vi "Menu Refs.vi"(8 "error in":errorcluster, 10 "Disabled 2":T1(ring), 11 "ATM Data":T2={"UI Refs"={"Right Buttons"=refnum, "Left Buttons"=refnum, "User Input"=refnum, "ATM Messages"=refnum, "Left Menu"=refnum, "Right Menu"=refnum, "Enter"=refnum}, "Map"={}, "Login Valid?"=FALSE, "Queue Message"=refnum, "State"=enum."None", "User"={"Pin"="", "First Name"="", "Last Name"="", "Balance"=0.0, "Login Valid?"=FALSE}, "Main States"={"Message"="Initialize", "Data"=variant}}) -> (0 "error out":errorcluster, 3 "ATM Data Out":T2={"UI Refs"={"Right Buttons"=refnum, "Left Buttons"=refnum, "User Input"=refnum, "ATM Messages"=refnum, "Left Menu"=refnum, "Right Menu"=refnum, "Enter"=refnum}, "Map"={}, "Login Valid?"=FALSE, "Queue Message"=refnum, "State"=enum."None", "User"={"Pin"="", "First Name"="", "Last Name"="", "Balance"=0.0, "Login Valid?"=FALSE}, "Main States"={"Message"="Initialize", "Data"=variant}})   [LabVIEW 2020, in "ATM Machine.lvlib"]
uses:
  ATM Machine.lvlib
  Cluster - ATM Machine Data.ctl
  Cluster - Message Cluster.ctl
  Enum - ATM States.ctl
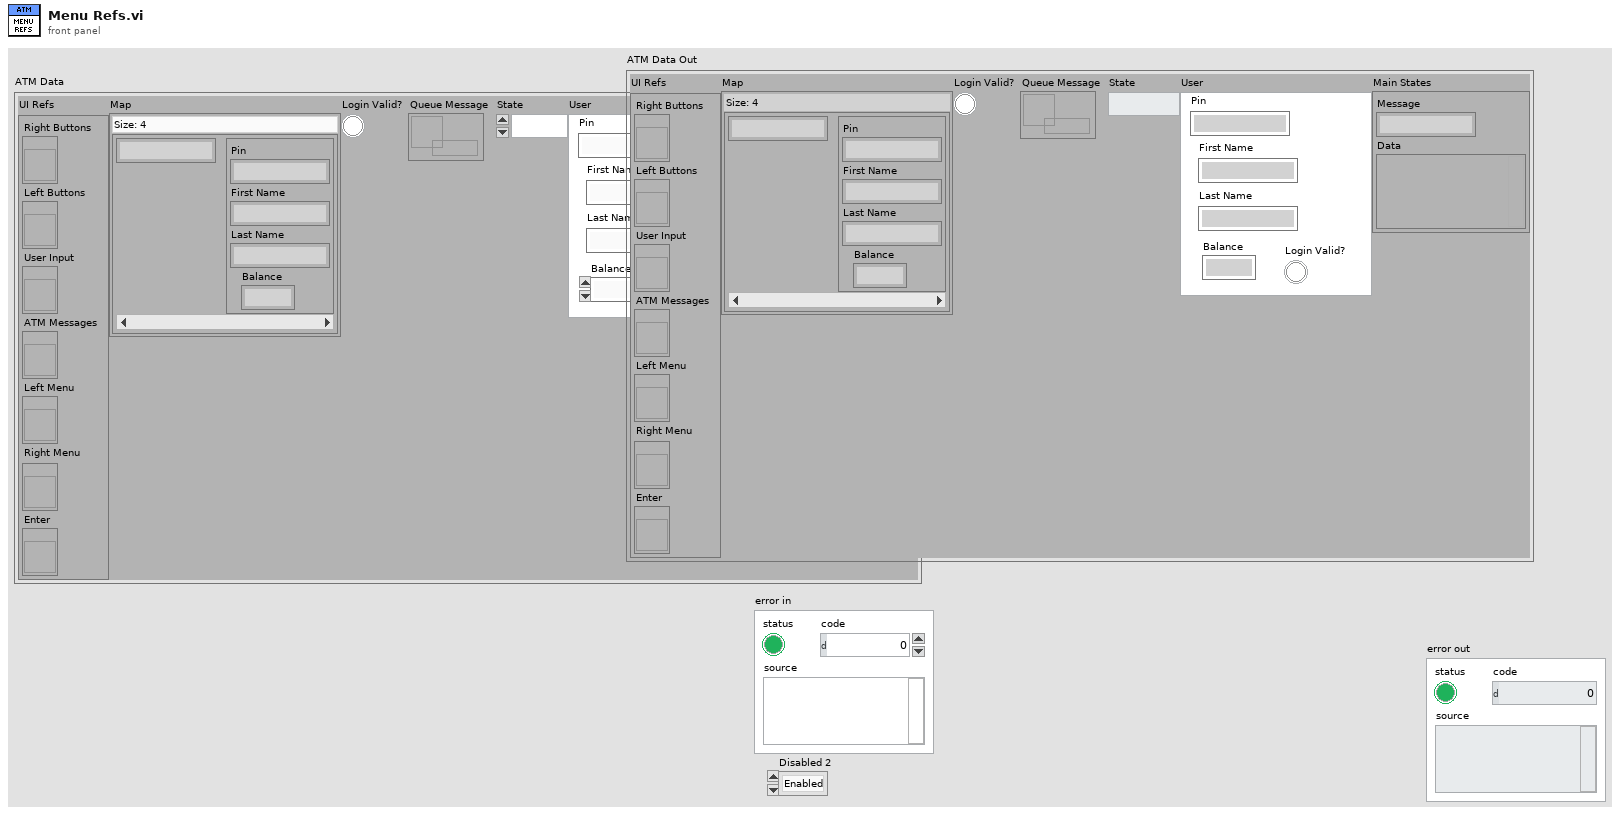
[diagram p1: front panel]
types:
  T1 = enum8{"Enabled", "Disabled", "Disabled and Grayed Out"}
  T2 = typedef "ATM Machine.lvlib/Cluster - ATM Machine Data.ctl" = cluster{"UI Refs":cluster{"Right Buttons":refnum<vi>, "Left Buttons":refnum<vi>, "User Input":refnum<vi>, "ATM Messages":refnum<vi>, "Left Menu":refnum<vi>, "Right Menu":refnum<vi>, "Enter":refnum<vi>}, "Map":map{string, cluster{"Pin":string, "First Name":string, "Last Name":string, "Balance":dbl}}, "Login Valid?":bool, "Queue Message":refnum<queue>, "State":T3, "User":cluster{"Pin":string, "First Name":string, "Last Name":string, "Balance":dbl, "Login Valid?":bool}, "Main States":cluster{"Message":string, "Data":variant}}
  T3 = typedef "ATM Machine.lvlib/Enum - ATM States.ctl" = enum16{"None", "Deposit", "Withdraw", "Card Inserted", "Balance Inquiry", "Return Card and Terminate", "Fast Cash"}
  T4 = cluster{"RFS String":string, "RFS String 2":string, "RFS String 3":string}
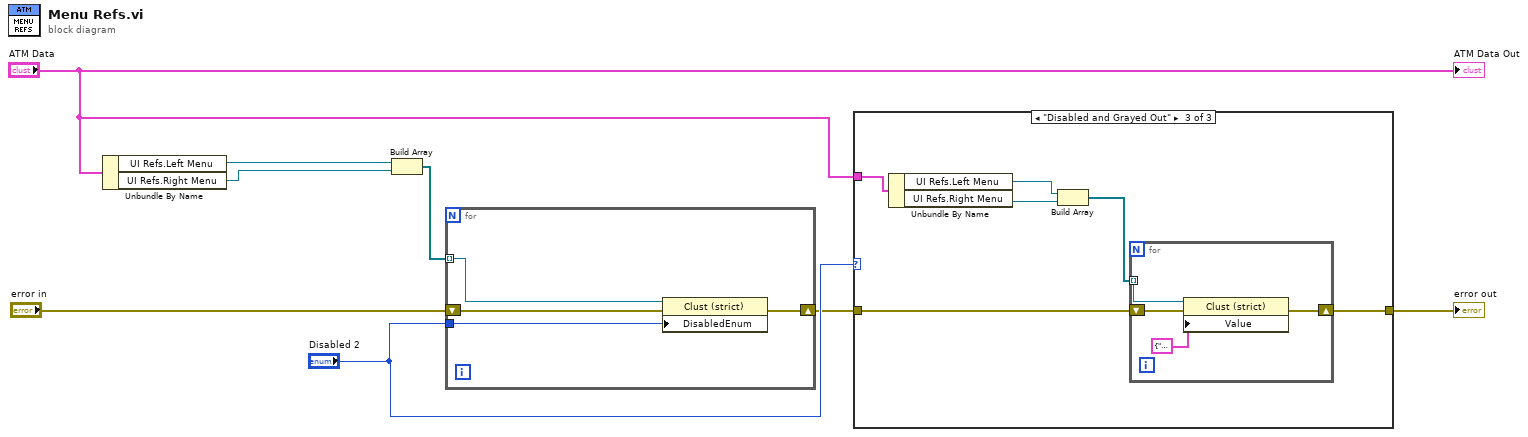
[diagram p0: block diagram]
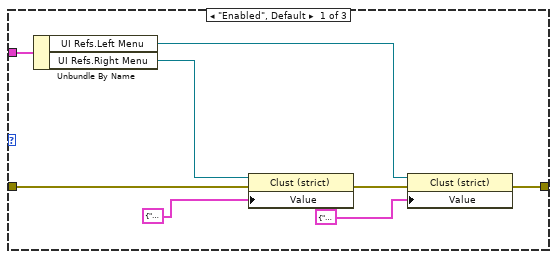
[diagram p2: hidden frame]
diagram:
  n1 = Unbundle By Name("ATM Data") -> ("UI Refs.Left Menu"=w6:refnum<vi>, "UI Refs.Right Menu"=w8:refnum<vi>)
  n2 = Build Array(w6, w8) -> (w7:refnum<vi>[])
  n3 = for {
    shift-right: [w11] -> w3
    shift-left: "error in" -> [w12]
    tunnel: w7 -> [w10] mode=indexing
    tunnel: "Disabled 2" -> [w9]
    n4 = property class="Clust (strict)"(reference=w10, error in=w12, "DisabledEnum"=w9) -> (error out=w11:errorcluster)  [unwired: 1 out]
  }
  n5 = case shown="\"Disabled and Grayed Out\"" "Disabled 2" {
    tunnel: [w19 w21 w27] -> w4
    tunnel: w3 -> [w15 w21 w22]
    tunnel: "ATM Data" -> [w20 _ w26]
    frame "Enabled", Default {
      n6 = Unbundle By Name(w20) -> ("UI Refs.Left Menu"=w18:refnum<vi>, "UI Refs.Right Menu"=w14:refnum<vi>)
      n7 = property class="Clust (strict)"(reference=w14, error in=w15, "Value"=T4 {"RFS String"="Deposit", "RFS String 2"="Withdrawal", "RFS String 3"="Fast Cash\n $50"} ("Right Menu")) -> (error out=w16:errorcluster)  [unwired: 1 out]
      n8 = property class="Clust (strict)"(reference=w18, error in=w16, "Value"=T4 {"RFS String"="None", "RFS String 2"="Balance Inquiry", "RFS String 3"="Return Card & Terminate"} ("Left Menu")) -> (error out=w19:errorcluster)  [unwired: 1 out]
    }
    frame "Disabled" {
    }
    frame "Disabled and Grayed Out" {
      n9 = Unbundle By Name(w26) -> ("UI Refs.Left Menu"=w25:refnum<vi>, "UI Refs.Right Menu"=w24:refnum<vi>)
      n10 = Build Array(w25, w24) -> (w23:refnum<vi>[])
      n11 = for {
        shift-right: [w30] -> w27
        shift-left: w22 -> [w29]
        tunnel: w23 -> [w28] mode=indexing
        n12 = property class="Clust (strict)"(reference=w28, error in=w29, "Value"=T4 {"RFS String"="", "RFS String 2"="", "RFS String 3"=""} ("Left Menu")) -> (error out=w30:errorcluster)  [unwired: 1 out]
      }
    }
  }
  "error out" <- w4
  "ATM Data Out" <- "ATM Data"
